vi "Close.vi"(11 "FpgaRefBase In":refnum<class "FpgaRefBase.lvclass">) -> ()   [LabVIEW 2018, in "FpgaRefBase.lvclass"]
uses:
  FpgaRefBase.lvclass
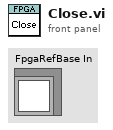
[diagram p1: front panel]
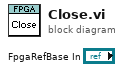
[diagram p0: block diagram]
diagram:
